vi "Auto AVG.vi"(8 "error in":errorcluster, 11 "All Input Tasks in":T1) -> (0 "error out":errorcluster, 1 "All Inputs cluster":T2, 3 "All Input Tasks out":T1)   [LabVIEW 2017]
uses:
  controls/All Inputs.ctl
  controls/SACB DI.ctl
  <vilib>/DAQmx/read.llb/DAQmx Read (Digital 1D Bool NChan 1Samp 1Line).vi
  <vilib>/DAQmx/read.llb/DAQmx Read (Counter DBL 1Chan 1Samp).vi
  <vilib>/DAQmx/read.llb/DAQmx Read (Analog 2D DBL NChan NSamp).vi
  GV/All Inputs.vi
  <vilib>/DAQmx/miscellaneous.llb/DAQmx Fill In Error Info.vi
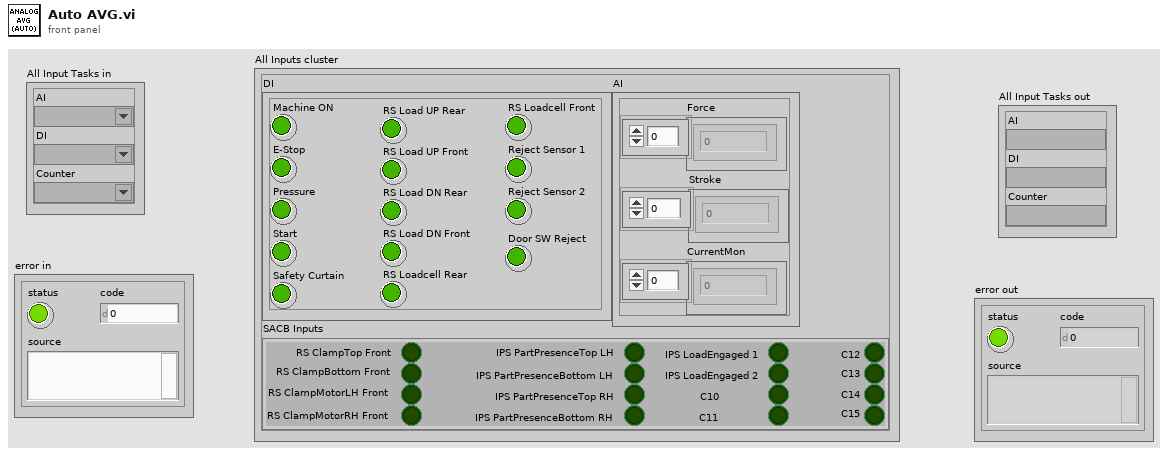
[diagram p1: front panel]
types:
  T1 = cluster{"AI":refnum<k21>, "DI":refnum<k21>, "Counter":refnum<k21>}
  T2 = typedef "All Inputs.ctl" = cluster{"DI":cluster{"Machine ON":bool, "E-Stop":bool, "Pressure":bool, "Start":bool, "Safety Curtain":bool, "RS Load UP Rear":bool, "RS Load UP Front":bool, "RS Load DN Rear":bool, "RS Load DN Front":bool, "RS Loadcell Rear":bool, "RS Loadcell Front":bool, "Reject Sensor 1":bool, "Reject Sensor 2":bool, "Door SW Reject":bool}, "AI":cluster{"Force":dbl[], "Stroke":dbl[], "CurrentMon":dbl[]}, "SACB Inputs":T3}
  T3 = typedef "SACB DI.ctl" = cluster{"RS ClampTop Front":bool, "RS ClampBottom Front":bool, "RS ClampMotorLH Front":bool, "RS ClampMotorRH Front":bool, "IPS PartPresenceTop LH":bool, "IPS PartPresenceBottom LH":bool, "IPS PartPresenceTop RH":bool, "IPS PartPresenceBottom RH":bool, "IPS LoadEngaged 1":bool, "IPS LoadEngaged 2":bool, "C10":bool, "C11":bool, "C12":bool, "C13":bool, "C14":bool, "C15":bool}
  T4 = cluster{"data[0]":bool, "data[1]":bool, "data[2]":bool, "data[3]":bool, "data[4]":bool, "data[5]":bool, "data[6]":bool, "data[7]":bool, "data[8]":bool, "data[9]":bool, "data[10]":bool, "data[11]":bool, "data[12]":bool, "data[13]":bool}
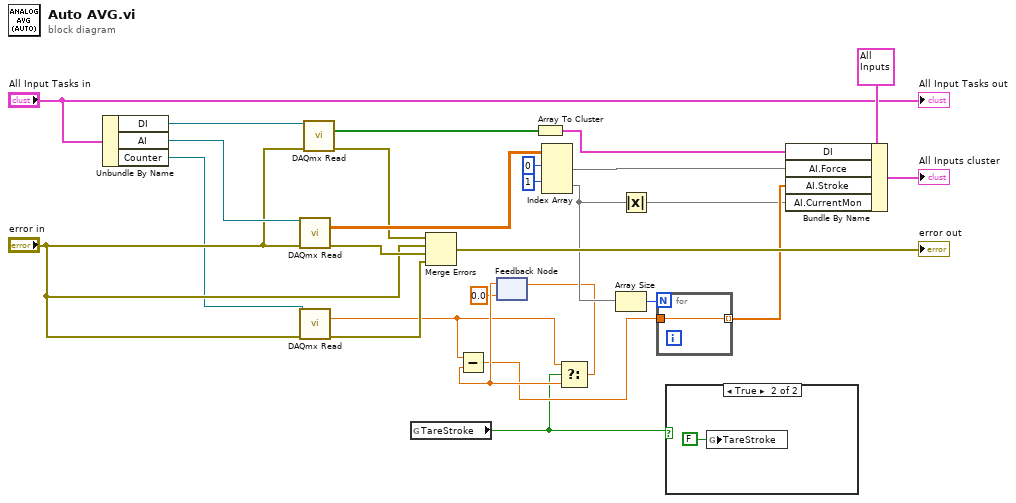
[diagram p0: block diagram]
diagram:
  n1 = Unbundle By Name("All Input Tasks in") -> ("DI"=w18:refnum<k21>, "AI"=w20:refnum<k21>, "Counter"=w8:refnum<k21>)
  n2 = call-poly <vilib>:"DAQmx Read.vi"("task/channels in"=w20, "error in"="error in") -> ("data"=w25:dbl[][], "error out"=w24:errorcluster)  [unwired: 11 in, 1 out]
  n3 = call-poly <vilib>:"DAQmx Read.vi"("task/channels in"=w8, "error in"="error in") -> ("data"=w5:dbl, "error out"=w14:errorcluster)  [unwired: 11 in, 1 out]
  n4 = call-poly <vilib>:"DAQmx Read.vi"("task/channels in"=w18, "error in"="error in") -> ("data"=w10:bool[], "error out"=w16:errorcluster)  [unwired: 11 in, 1 out]
  n5 = global read "All Inputs.vi" "TareStroke"() -> (w2:bool)
  n6 = Merge Errors(w16, "error in", w24, w14) -> (→"error out":errorcluster)
  n7 = feedback #1(0.0 ("data")) -> (w7:dbl)
  n8 = Subtract(x=w5, y=w7) -> (x-y=w4:dbl)
  n9 = Array To Cluster(array=w10) -> (cluster=w19:T4)
  n10 = Index Array(array=w25, index (row) #1=0, index (row) #2=1) -> (element #1=w9:dbl[], element #2=w11:dbl[])  [unwired: 2 in]
  n11 = Select(t=w5, s=w2, f=w7) -> (s? t:f=w6:dbl)
  n12 = feedback-in #1(w6) -> ()
  n13 = Array Size(array=w11) -> (size(s)=w12:i32)
  n14 = Absolute Value(x=w11) -> (abs(x)=w1:dbl[])
  n15 = for {
    N: w12 -> [_]
    tunnel: w4 -> [w28]
    tunnel: [w28] -> w13 mode=indexing
  }
  n16 = case shown="True" w2 {
    frame False {
    }
    frame True {
      n17 = global write "All Inputs.vi" "TareStroke"(FALSE ("TareStroke")) -> ()
    }
  }
  n18 = Bundle By Name(cluster=T2 {"DI"={"Machine ON"=FALSE, "E-Stop"=FALSE, "Pressure"=FALSE, "Start"=FALSE, "Safety Curtain"=FALSE, "RS Load UP Rear"=FALSE, "RS Load UP Front"=FALSE, "RS Load DN Rear"=FALSE, "RS Load DN Front"=FALSE, "RS Loadcell Rear"=FALSE, "RS Loadcell Front"=FALSE, "Reject Sensor 1"=FALSE, "Reject Sensor 2"=FALSE, "Door SW Reject"=FALSE}, "AI"={"Force"=[], "Stroke"=[], "CurrentMon"=[]}, "SACB Inputs"={"RS ClampTop Front"=FALSE, "RS ClampBottom Front"=FALSE, "RS ClampMotorLH Front"=FALSE, "RS ClampMotorRH Front"=FALSE, "IPS PartPresenceTop LH"=FALSE, "IPS PartPresenceBottom LH"=FALSE, "IPS PartPresenceTop RH"=FALSE, "IPS PartPresenceBottom RH"=FALSE, "IPS LoadEngaged 1"=FALSE, "IPS LoadEngaged 2"=FALSE, "C10"=FALSE, "C11"=FALSE, "C12"=FALSE, "C13"=FALSE, "C14"=FALSE, "C15"=FALSE}} ("Inputs"), "DI"=w19, "AI.Force"=w9, "AI.Stroke"=w13, "AI.CurrentMon"=w1) -> (→"All Inputs cluster":T2)
  "All Input Tasks out" <- "All Input Tasks in"
